vi "simple test.vi"() -> ()   [LabVIEW 2019, in "Inst.RP100.lvlib" / "Inst.RP100.lvclass"]
uses:
  Inst.RP100.lvclass
  C:/Program Files (x86)/National Instruments/LabVIEW 2019/user.lib/LevyLab/Instrument Framework/Instrument/Instrument.lvclass
  <userlib>/LevyLab/Instrument Framework/Instrument/Instrument.lvclass/Instrument.ctl
  <userlib>/LevyLab/Instrument Framework/Instrument/Instrument.lvclass
panel:
  in  "VISA resource name":refnum<visa-resource-name>
  out "error out":errorcluster
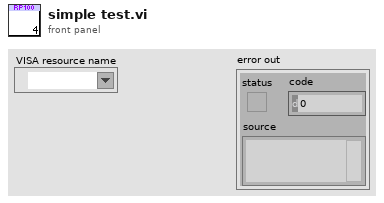
[diagram p1: front panel]
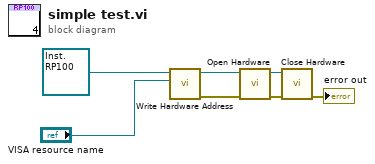
[diagram p0: block diagram]
diagram:
  n1 = call <userlib>:"Write Hardware Address.vi"("Address"="VISA resource name", "Instrument in"=refnum<class "Inst.RP100.lvclass"> refnum ("Inst.RP100.lvlib:Inst.RP100.lvclass")) -> ("error out"=w1:errorcluster, "Instrument out"=w3:refnum<class "Inst.RP100.lvclass">)  [unwired: 8 in]
  n2 = call-dynamic "Open Hardware.vi"("error in (no error)"=w1, "Inst.RP100 in"=w3) -> ("error out"=w6:errorcluster, "Inst.RP100 out"=w7:refnum<class "Inst.RP100.lvclass">)  [unwired: 8 in]
  n3 = call-dynamic "Close Hardware.vi"("error in (no error)"=w6, "Inst.RP100 in"=w7) -> ("error out"=→"error out":errorcluster)  [unwired: 8 in, 1 out]
